vi "Node Archive and FTP File Handler.vi"() -> ()   [LabVIEW 2010]
doc: "NODE ARCHIVE & FTP is a software used to handle the file management of remote field sites using the HTI Data Logger or ATR series acoustic equipment that generates *.RAT and *.ATL files. The software monitors a specific folder on the local machine that the HTI equipment has been set up to move completed files of these types into. All other file types are ignored. The software continues to scan this file until a new file is added to the directory, on the addition of a file the NODE ARCHIVE & FTP software moves the file into an Archive directory (and if specified into a redundant Archive directory) then creates a *.ZIP version of the file and retains a copy of it in the Archive directory as well. All Zip files are then copied to a specified FTP host.\n\nNODE ARCHIVE & FTP will not try and move files for the last five minutes of an hour, or for the first five to ten minutes of the hour (based on CPU time). This is to allow the HTI hardware time to move all files at the top of the hour and avoid conflict. During the rest of the hour the software will continue to scan for new files. At any time a user can force a scan or FTP move by selecting the Manual Force FTP button or the Manual Archive Files button.\n\nNODE ARCHIVE & FTP creates an .INI file and a .CSV file in the programs application directory. The .INI file retains the last values of the file directory and FTP credentials used. The .CSV retains a history of *.ZIP files moved to the FTP and the status of their move, if there were errors or not. NODE ARCHIVE & FTP will continue to try and send the file to the FTP host until that file has completed the process with no errors. DO NOT remove or edit the .CSV file or the software will try and move all files up to the FTP again and will slow down the FTP Host."
uses:
  FTP Credintials.ctl
  <vilib>/Utility/sysdir.llb/System Directory Type.ctl
  <vilib>/Utility/error.llb/DialogType.ctl
  <vilib>/Utility/config.llb/Read Key (String).vi
  <vilib>/Utility/config.llb/Read Key (Boolean).vi
  <vilib>/Utility/config.llb/Read Key (Path).vi
  <vilib>/Utility/config.llb/Read Key (I32).vi
  <vilib>/Utility/config.llb/Write Key (Path).vi
  <vilib>/Utility/config.llb/Write Key (Boolean).vi
  <vilib>/Utility/config.llb/Write Key (String).vi
  <vilib>/Utility/config.llb/Write Key (I32).vi
  <vilib>/Utility/config.llb/NI_LVConfig.lvlib
  Aarons labview builds/telemetryCode/Utilities/NewNI_SMTPEmail Folder/NewNI_SMTPEmail.lvlib
panel:
  in  "Time DaY":timestamp
  in  "Top level Tabs":T1(tab)
  in  "ShutDown":bool
  out "Status File move":bool caption="Archiving"
  out "Status FTP move":bool caption="FTP In Progress"
  in  "Manual FTP":bool
  in  "Manual Archive":bool
  in  "FTP Creds":T2 {"FTP Timeout (S)" min=0 max=300 step=1}
  in  "Archive Location 2":path caption="(Optional) External Directory To Archive *.RAT files"
  in  "Archive Location":path=path "C:/Archive" caption="Directory To Archive *.RAT files"
  in  "Rats Location":path=path "C:/Incoming" caption="Directory To Find *.RAT files"
  in  "Ping FTP Host":bool=TRUE
  in  "Ping Node 2":bool=TRUE
  in  "Ping Node 1":bool=TRUE
  out "Node 2 Response":bool
  in  "AddressNode2":string="www.google.com" caption="Address of Node 2 to Ping"
  out "FTP Response":bool
  out "Node1 Response":bool
  in  "recipients":string[](array[string])=["nmswyers@gmail.com"] caption="Email Recipients"
  in  "Addresshost":string="50.6.185.144" caption="Address of FTP host to Ping"
  in  "AddressNode 1":string="www.google.com" caption="Address of Node 1 to Ping"
  out "Elapsed Time (H)":dbl caption="Time to Next File \nSize Check (H)" format="%#_3f"
  out "Email Notification":T3 caption="Email Notification (From INI File)"
  # "DIRECTORY SETUP:"
  # "FTP SETUP:"
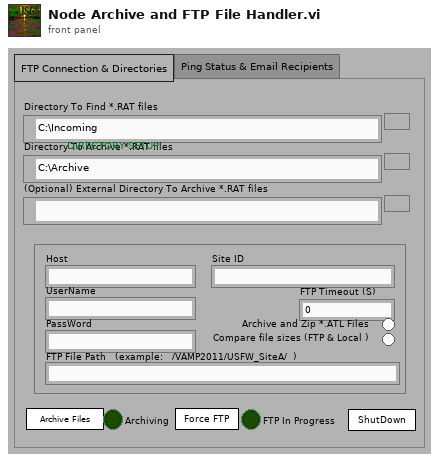
[diagram p1: front panel]
types:
  T1 = enum32{"FTP Connection & Directories", "Ping Status & Email Recipients"}
  T2 = typedef "FTP Credintials.ctl" = cluster{"Host":string, "UserName":string, "PassWord":string, "FTP File Path":string, "FTP Timeout (S)":i32, "Use ATL":bool, "Comp File Size":bool, "SITE ID":string}
  T3 = cluster{"Mail Server":string, "Return Address":string, "User Name":string, "Password":string}
  T4 = cluster{"Mail Server":string, "Return Address":string, "Email User Name":string, "Password":string}
  T5 = typedef "System Directory Type.ctl" = i32
  T6 = typedef "NI_LVConfig.lvlib/Config Data RefNum.ctl" = refnum<k1>
  T7 = typedef "DialogType.ctl" = u16
  T8 = cluster{"AddressNode 1":string, "AddressNode2":string, "Addresshost":string}
  T9 = enum16{"open", "replace", "create", "open or create", "replace or create", "replace or create with confirmation"}
  T10 = enum32{"invalid app kind", "Development System", "Run Time System", "Student Edition", "Embedded LabVIEW", "Evaluation", "Custom"}
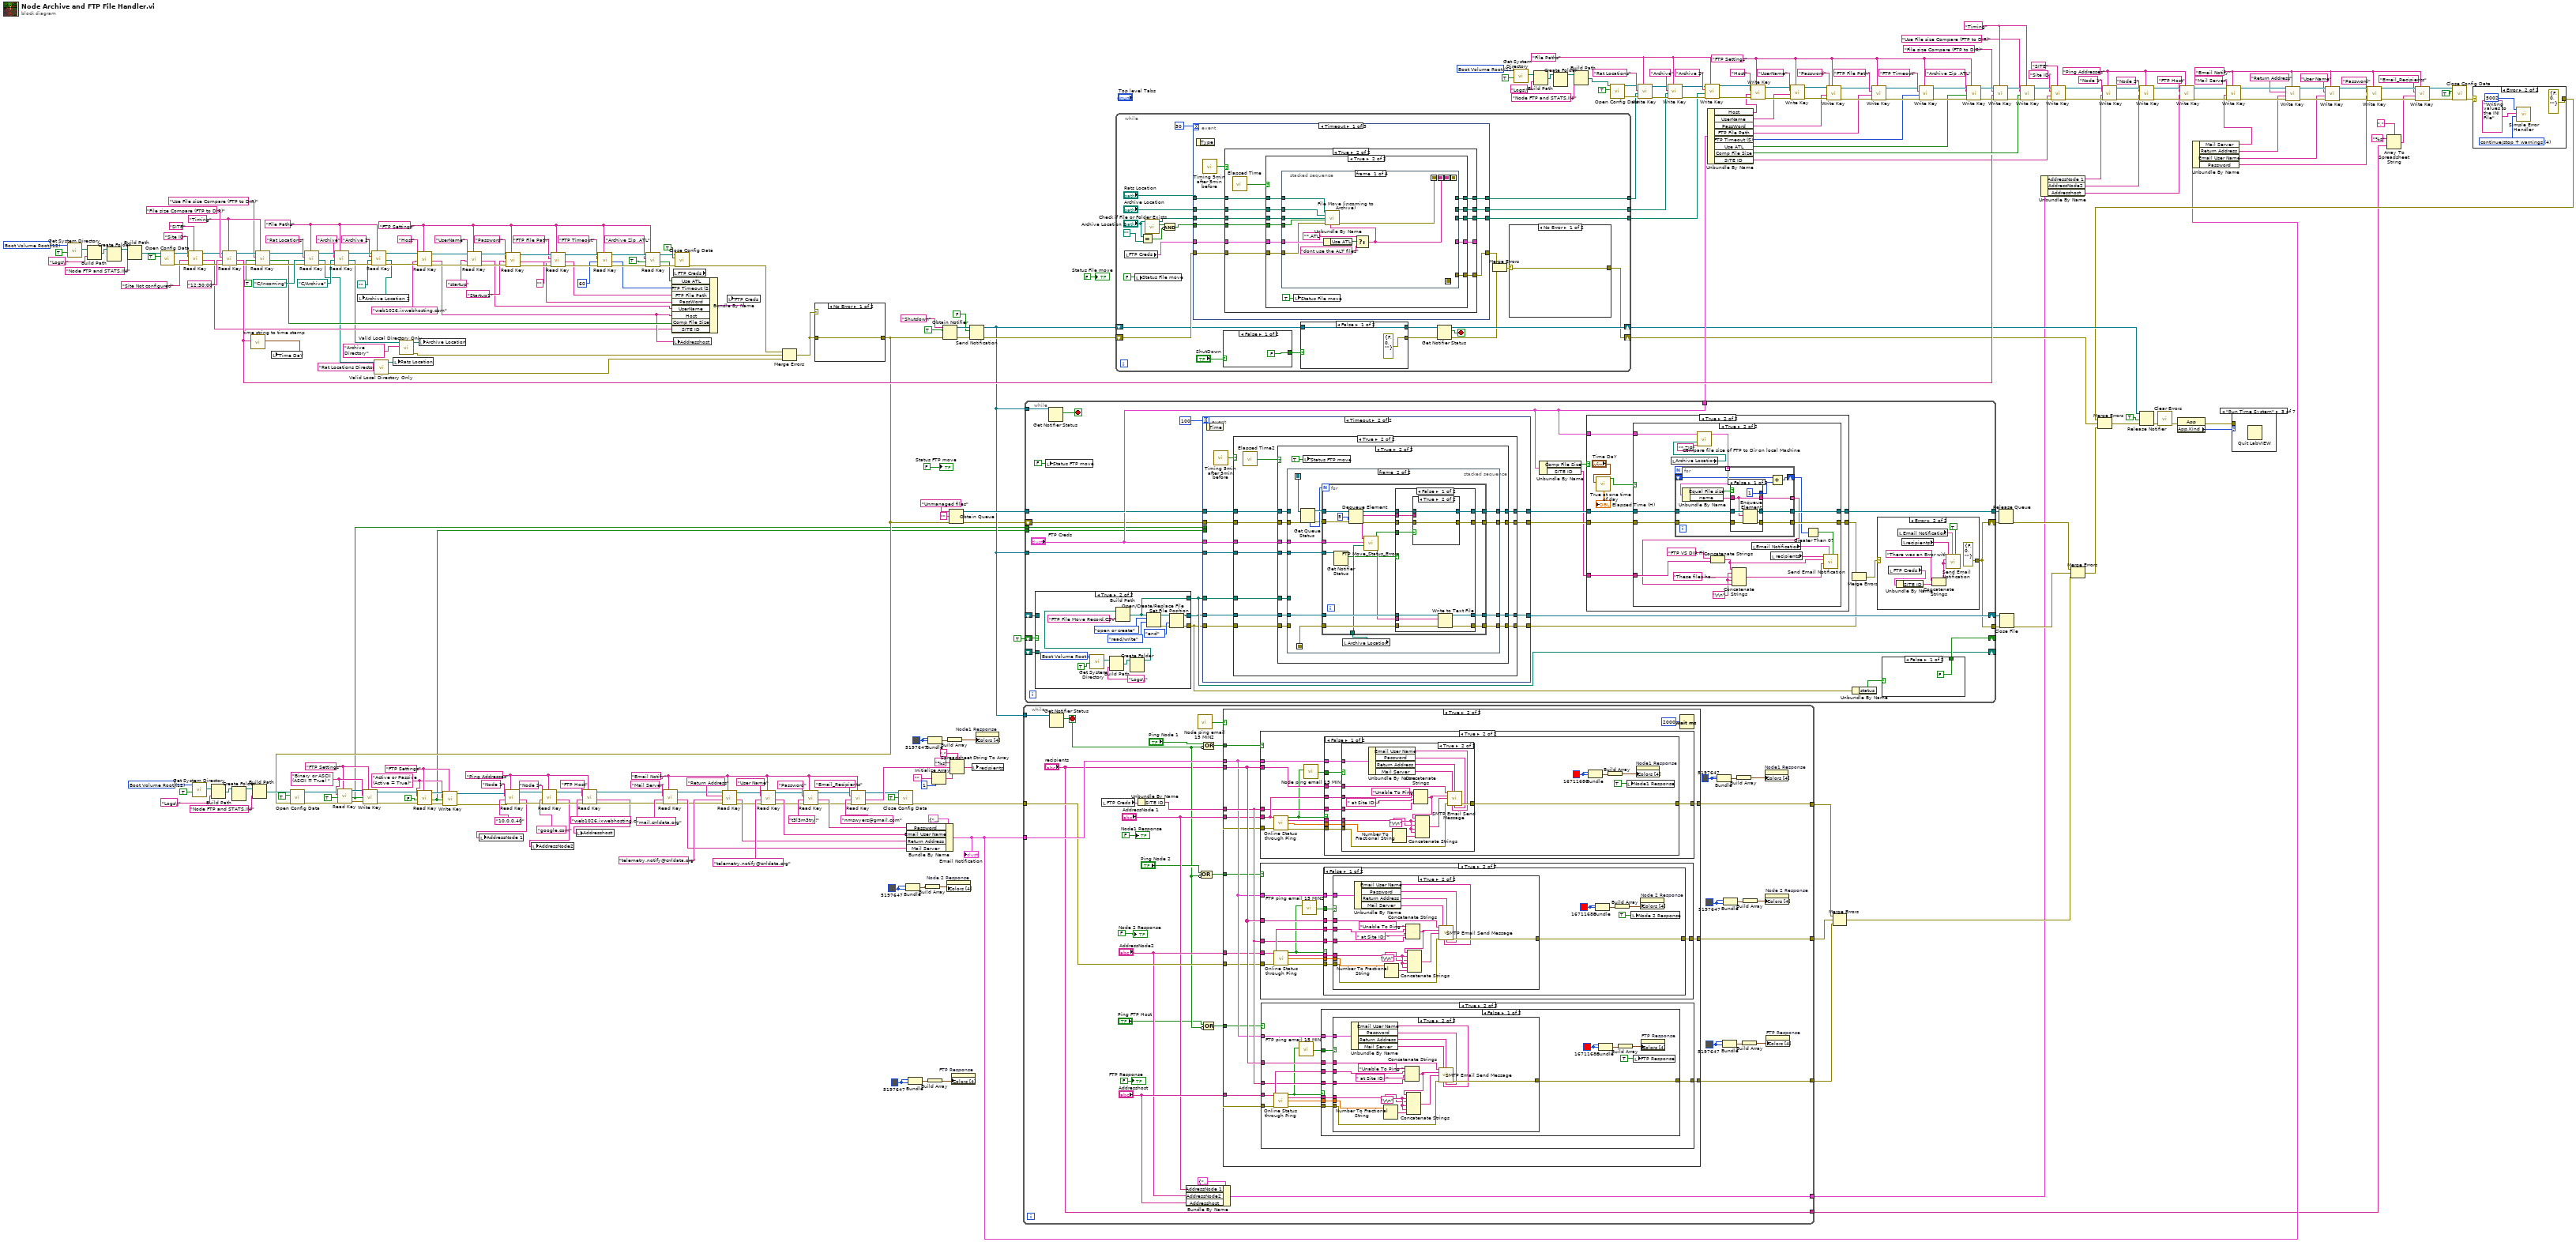
[diagram p0: block diagram]
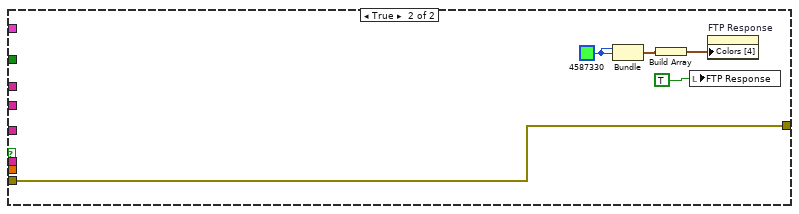
[diagram p5: hidden frame]
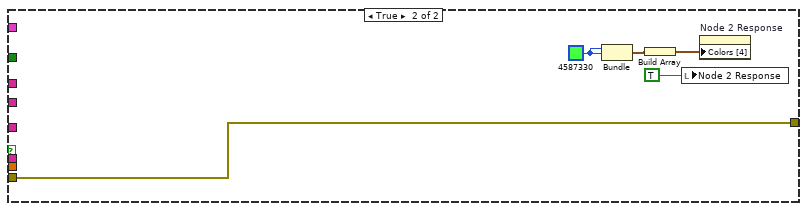
[diagram p8: hidden frame]
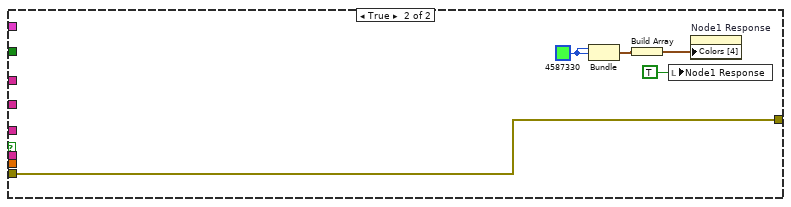
[diagram p11: hidden frame]
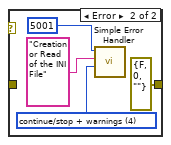
[diagram p13: hidden frame]
diagram:
  w2 = "Email Notify" ("name or relative path")
  w57 = "Binary or ASCII (ASCII = True) " ("name or relative path")
  w56 = "FTP Settings" ("name or relative path")
  w63 = "Active or Passive (Active = True)" ("name or relative path")
  w64 = "FTP Settings" ("name or relative path")
  w80 = "Ping Addresses" ("name or relative path")
  w93 = "Ping Addresses" ("name or relative path")
  w129 = u32 5197647 ("Color Box")
  w1 = "Email Notify" ("name or relative path")
  w139 = T5 12 items=["User Home"=0, "User Desktop"=1, "User Documents"=2, "User Application Data"=3, "User Preferences"=4, "User Temporary"=5, "Public Documents"=6, "Public Application Data"=7, "Public Preferences"=8, "Public Cache"=13, "System Core Libraries"=9, "System Installed Libraries"=10, "Application Files"=11, "Boot Volume Root"=12] ("system directory type")
  w155 = T5 12 items=["User Home"=0, "User Desktop"=1, "User Documents"=2, "User Application Data"=3, "User Preferences"=4, "User Temporary"=5, "Public Documents"=6, "Public Application Data"=7, "Public Preferences"=8, "Public Cache"=13, "System Core Libraries"=9, "System Installed Libraries"=10, "Application Files"=11, "Boot Volume Root"=12] ("system directory type")
  w193 = u32 5197647 ("Color Box")
  w190 = u32 5197647 ("Color Box")
  w201 = "Timing" ("name or relative path")
  w211 = "Timing" ("name or relative path")
  w266 = "FTP Settings" ("name or relative path")
  w250 = "File Paths" ("name or relative path")
  w286 = "FTP Settings" ("name or relative path")
  w304 = "File Paths" ("name or relative path")
  w306 = T5 12 items=["User Home"=0, "User Desktop"=1, "User Documents"=2, "User Application Data"=3, "User Preferences"=4, "User Temporary"=5, "Public Documents"=6, "Public Application Data"=7, "Public Preferences"=8, "Public Cache"=13, "System Core Libraries"=9, "System Installed Libraries"=10, "Application Files"=11, "Boot Volume Root"=12] ("system directory type")
  n1 = call <vilib>:"Get System Directory.vi"("create directory if not found? (F)"=TRUE, "system directory type"=w306) -> ("system directory"=w307:path)  [unwired: 9 in]
  n2 = Build Path(base path=w307, name or relative path="Logs\\" ("string")) -> (appended path=w165:path)
  n3 = Create Folder(path (use dialog)=w165) -> (created path=w164:path)  [unwired: 2 in, 2 out]
  n4 = Build Path(base path=w164, name or relative path="Node FTP and STATS.INI") -> (appended path=w162:path)
  n5 = call <vilib>:"Open Config Data.vi"("create file if necessary (T)"=TRUE, "configuration file path"=w162) -> ("error out"=w188:errorcluster, "refnum"=w187:T6)  [unwired: 7 in, 1 out]
  n6 = call-poly <vilib>:"Read Key.vi"("section"="SITE" ("name or relative path"), "error in (no error)"=w188, "default value"="Site Not configured", "key"="Site ID" ("name or relative path"), "refnum"=w187) -> ("error out"=w185:errorcluster, "value"=w181:string, "refnum out"=w186:T6)  [unwired: 3 in, 1 out]
  n7 = call <vilib>:"Get System Directory.vi"("create directory if not found? (F)"=TRUE, "system directory type"=w139) -> ("system directory"=w138:path)  [unwired: 9 in]
  n8 = Build Path(base path=w138, name or relative path="Logs\\" ("string")) -> (appended path=w144:path)
  n9 = call-poly <vilib>:"Read Key.vi"("section"=w211, "error in (no error)"=w185, "default value"="12:30:00", "key"="File size Compare (FTP to DIR)" ("name or relative path"), "refnum"=w186) -> ("error out"=w215:errorcluster, "value"=w196:string, "refnum out"=w214:T6)  [unwired: 3 in, 1 out]
  n10 = Create Folder(path (use dialog)=w144) -> (created path=w145:path)  [unwired: 2 in, 2 out]
  n11 = call "time string to time stamp.vi"("time string example(16:15:00)"=w196) -> ("time stamp"=w208:timestamp)  [unwired: 10 in]
  n12 = Build Path(base path=w145, name or relative path="Node FTP and STATS.INI") -> (appended path=w147:path)
  n13 = call-poly <vilib>:"Read Key.vi"("section"=w211, "error in (no error)"=w215, "default value"=TRUE ("create file if necessary (T)"), "key"="Use File size Compare (FTP to DIR)" ("name or relative path"), "refnum"=w214) -> ("error out"=w212:errorcluster, "value"=w198:bool, "refnum out"=w213:T6)  [unwired: 3 in, 1 out]
  n14 = local write "Time DaY"(w208) -> ()
  n15 = call-poly <vilib>:"Read Key.vi"("section"=w304, "error in (no error)"=w212, "default value"=path "C:/Incoming", "key"="Rat Locations" ("name or relative path"), "refnum"=w213) -> ("error out"=w311:errorcluster, "value"=w174:path, "refnum out"=w312:T6)  [unwired: 3 in, 1 out]
  n16 = call-poly <vilib>:"Read Key.vi"("section"=w304, "error in (no error)"=w311, "default value"=path "C:/Archive", "key"="Archive" ("name or relative path"), "refnum"=w312) -> ("error out"=w309:errorcluster, "value"=w170:path, "refnum out"=w310:T6)  [unwired: 3 in, 1 out]
  n17 = call-poly <vilib>:"Read Key.vi"("section"=w304, "error in (no error)"=w309, "default value"=path "", "key"="Archive 2" ("name or relative path"), "refnum"=w310) -> ("error out"=w300:errorcluster, "value"=w161:path, "refnum out"=w293:T6)  [unwired: 3 in, 1 out]
  n18 = local write "Archive Location 2"(w161) -> ()
  n19 = call "Valid Local Directory Only.vi"("Directory ref"="Rat Locations Directory", "Path input"=w174) -> ("error out"=w149:errorcluster, "Path output"=w172:path)  [unwired: 8 in]
  n20 = local write "Rats Location"(w172) -> ()
  n21 = call "Valid Local Directory Only.vi"("Directory ref"="Archive Directory", "Path input"=w170) -> ("error out"=w150:errorcluster, "Path output"=w169:path)  [unwired: 8 in]
  n22 = call-poly <vilib>:"Read Key.vi"("section"=w286, "error in (no error)"=w300, "default value"="web1026.ixwebhosting.com" ("name or relative path"), "key"="Host" ("name or relative path"), "refnum"=w293) -> ("error out"=w299:errorcluster, "value"=w194:string, "refnum out"=w292:T6)  [unwired: 3 in, 1 out]
  n23 = local write "Archive Location"(w169) -> ()
  n24 = call-poly <vilib>:"Read Key.vi"("section"=w286, "error in (no error)"=w299, "default value"="startup" ("name or relative path"), "key"="UserName" ("name or relative path"), "refnum"=w292) -> ("error out"=w298:errorcluster, "value"=w230:string, "refnum out"=w291:T6)  [unwired: 3 in, 1 out]
  n25 = call-poly <vilib>:"Read Key.vi"("section"=w286, "error in (no error)"=w298, "default value"="Startup1" ("name or relative path"), "key"="Password" ("name or relative path"), "refnum"=w291) -> ("error out"=w297:errorcluster, "value"=w231:string, "refnum out"=w290:T6)  [unwired: 3 in, 1 out]
  n26 = call-poly <vilib>:"Read Key.vi"("section"=w286, "error in (no error)"=w297, "default value"="" ("name or relative path"), "key"="FTP File Path" ("name or relative path"), "refnum"=w290) -> ("error out"=w296:errorcluster, "value"=w232:string, "refnum out"=w289:T6)  [unwired: 3 in, 1 out]
  n27 = call-poly <vilib>:"Read Key.vi"("section"=w286, "error in (no error)"=w296, "default value"=60, "key"="FTP Timeout" ("name or relative path"), "refnum"=w289) -> ("error out"=w295:errorcluster, "value"=w67:i32, "refnum out"=w288:T6)  [unwired: 3 in, 1 out]
  n28 = call-poly <vilib>:"Read Key.vi"("section"=w286, "error in (no error)"=w295, "default value"=TRUE, "key"="Archive Zip .ATL" ("name or relative path"), "refnum"=w288) -> ("error out"=w294:errorcluster, "value"=w233:bool, "refnum out"=w287:T6)  [unwired: 3 in, 1 out]
  n29 = local read "FTP Creds"() -> (w234:T2)
  n30 = Bundle By Name(cluster=w234, "Use ATL"=w233, "FTP Timeout (S)"=w67, "FTP File Path"=w232, "PassWord"=w231, "UserName"=w230, "Host"=w194, "Comp File Size"=w198, "SITE ID"=w181) -> (w235:T2)
  n31 = local write "Addresshost"(w194) -> ()
  n32 = call <vilib>:"Close Config Data.vi"("error in (no error)"=w294, "write file if changed (T)"=TRUE, "refnum"=w287) -> ("error out"=w151:errorcluster)  [unwired: 7 in, 1 out]
  n33 = local write "FTP Creds"(w235) -> ()
  n34 = Merge Errors(w151, w150, w149) -> (w152:errorcluster)
  n35 = case shown="No Error" w152 {
    tunnel: w152 -> [w314 _]
    tunnel: [w314 errorcluster {"status"=FALSE, "code"=0, "source"=""} ("error out")] -> w104
    frame No Error {
    }
    frame Error {
      w318 = T7 4 items=["no dialog", "OK message", "continue or stop message", "OK message + warnings", "continue/stop + warnings"] ("type of dialog (OK msg:1)")
      n36 = call <vilib>:"Simple Error Handler.vi"("error code (no error:0)"=5001, "error source (\" \")"="Creation or Read of the INI File" ("error source (\" \")"), "type of dialog (OK msg:1)"=w318) -> ()  [unwired: 2 in, 5 out]
    }
  }
  n37 = call <vilib>:"Open Config Data.vi"("error in (no error)"=w104, "create file if necessary (T)"=TRUE, "configuration file path"=w147) -> ("error out"=w53:errorcluster, "refnum"=w54:T6)  [unwired: 6 in, 1 out]
  n38 = call-poly <vilib>:"Read Key.vi"("section"=w56, "error in (no error)"=w53, "default value"=TRUE, "key"=w57, "refnum"=w54) -> ("error out"=w52:errorcluster, "value"=w49:bool, "refnum out"=w55:T6)  [unwired: 3 in, 1 out]
  n39 = call-poly <vilib>:"Write Key.vi"("section"=w56, "error in (no error)"=w52, "value"=w49, "key"=w57, "refnum"=w55) -> ("error out"=w51:errorcluster, "refnum out"=w50:T6)  [unwired: 4 in, 1 out]
  n40 = call-poly <vilib>:"Read Key.vi"("section"=w64, "error in (no error)"=w51, "default value"=FALSE, "key"=w63, "refnum"=w50) -> ("error out"=w66:errorcluster, "value"=w59:bool, "refnum out"=w65:T6)  [unwired: 3 in, 1 out]
  n41 = call-poly <vilib>:"Write Key.vi"("section"=w64, "error in (no error)"=w66, "value"=w59, "key"=w63, "refnum"=w65) -> ("error out"=w60:errorcluster, "refnum out"=w61:T6)  [unwired: 4 in, 1 out]
  n42 = call-poly <vilib>:"Read Key.vi"("section"=w93, "error in (no error)"=w60, "default value"="10.0.0.40", "key"="Node 1" ("Mail Server"), "refnum"=w61) -> ("error out"=w91:errorcluster, "value"=w86:string, "refnum out"=w92:T6)  [unwired: 3 in, 1 out]
  n43 = local write "AddressNode 1"(w86) -> ()
  n44 = call-poly <vilib>:"Read Key.vi"("section"=w93, "error in (no error)"=w91, "default value"="google.com", "key"="Node 2" ("Mail Server"), "refnum"=w92) -> ("error out"=w90:errorcluster, "value"=w85:string, "refnum out"=w89:T6)  [unwired: 3 in, 1 out]
  n45 = local write "AddressNode2"(w85) -> ()
  n46 = call-poly <vilib>:"Read Key.vi"("section"=w93, "error in (no error)"=w90, "default value"="web1026.ixwebhosting.com", "key"="FTP Host" ("Mail Server"), "refnum"=w89) -> ("error out"=w87:errorcluster, "value"=w84:string, "refnum out"=w88:T6)  [unwired: 3 in, 1 out]
  n47 = local write "Addresshost"(w84) -> ()
  n48 = call-poly <vilib>:"Read Key.vi"("section"=w1, "error in (no error)"=w87, "default value"="mail.crrldata.org", "key"="Mail Server" ("Mail Server"), "refnum"=w88) -> ("error out"=w47:errorcluster, "value"=w118:string, "refnum out"=w46:T6)  [unwired: 3 in, 1 out]
  n49 = call-poly <vilib>:"Read Key.vi"("section"=w1, "error in (no error)"=w47, "default value"="telemetry.notify@crrldata.org", "key"="Return Address" ("Return Address"), "refnum"=w46) -> ("error out"=w45:errorcluster, "value"=w119:string, "refnum out"=w42:T6)  [unwired: 3 in, 1 out]
  n50 = call-poly <vilib>:"Read Key.vi"("section"=w1, "error in (no error)"=w45, "default value"="telemetry.notify@crrldata.org", "key"="User Name" ("Email User Name"), "refnum"=w42) -> ("error out"=w44:errorcluster, "value"=w120:string, "refnum out"=w43:T6)  [unwired: 3 in, 1 out]
  n51 = call-poly <vilib>:"Read Key.vi"("section"=w1, "error in (no error)"=w44, "default value"="t3l3m3try!", "key"="Password" ("Password"), "refnum"=w43) -> ("error out"=w33:errorcluster, "value"=w121:string, "refnum out"=w34:T6)  [unwired: 3 in, 1 out]
  n52 = call-poly <vilib>:"Read Key.vi"("section"=w1, "error in (no error)"=w33, "default value"="nmswyers@gmail.com", "key"="Email_Recipients" ("Password"), "refnum"=w34) -> ("error out"=w30:errorcluster, "value"=w32:string, "refnum out"=w31:T6)  [unwired: 3 in, 1 out]
  n53 = call <vilib>:"Close Config Data.vi"("error in (no error)"=w30, "write file if changed (T)"=TRUE, "refnum"=w31) -> ("error out"=w132:errorcluster)  [unwired: 7 in, 1 out]
  n54 = Bundle("Color Box"=w193, "Color Box"=w193) -> (w192:cluster{"Color Box":u32, "Color Box":u32})  [unwired: 1 in]
  n55 = Bundle By Name(cluster=T4 {"Mail Server"="Mail Server", "Return Address"="Return Address", "Email User Name"="User Name", "Password"="Password"} ("input cluster"), "Password"=w121, "Email User Name"=w120, "Return Address"=w119, "Mail Server"=w118) -> (w11:T4)
  "Email Notification" <- w11
  n56 = Bundle("Color Box"=w129, "Color Box"=w129) -> (w130:cluster{"Color Box":u32, "Color Box":u32})  [unwired: 1 in]
  n57 = Build Array(w192) -> (w128:cluster{"Color Box":u32, "Color Box":u32}[])
  n58 = Bundle("Color Box"=w190, "Color Box"=w190) -> (w189:cluster{"Color Box":u32, "Color Box":u32})  [unwired: 1 in]
  n59 = Build Array(w130) -> (w131:cluster{"Color Box":u32, "Color Box":u32}[])
  n60 = Initialize Array("", 1 ("dimension size")) -> (w41:string[])
  n61 = Obtain Notifier(name (unnamed)="Shutdown", notification data type=TRUE, error in (no error)=w104) -> (notifier out=w115:refnum<notifier>, error out=w113:errorcluster)  [unwired: 1 in, 1 out]
  n62 = property on="Node 2 Response" class="Bool (strict)"("Colors [4]"=w128) -> ()  [unwired: 2 in, 2 out]
  n63 = Build Array(w189) -> (w191:cluster{"Color Box":u32, "Color Box":u32}[])
  n64 = Obtain Queue(name (unnamed)="Unmanaged files", element data type="" ("name (unnamed)"), error in (no error)=w104) -> (queue out=w222:refnum<queue>, error out=w48:errorcluster)  [unwired: 2 in, 1 out]
  n65 = Spreadsheet String To Array(delimiter (Tab)=",", format string="%s", spreadsheet string=w32, array type (2D Dbl)=w41) -> (array=w29:string[])
  n66 = property on="FTP Response" class="Bool (strict)"("Colors [4]"=w131) -> ()  [unwired: 2 in, 2 out]
  n67 = Send Notification(notification=FALSE, notifier=w115, error in (no error)=w113) -> (notifier out=w68:refnum<notifier>, error out=w112:errorcluster)
  n68 = local write "recipients"(w29) -> ()
  n69 = property on="Node1 Response" class="Bool (strict)"("Colors [4]"=w191) -> ()  [unwired: 2 in, 2 out]
  n70 = while {
    tunnel: w132 -> [w342]
    tunnel: [w349] -> w168
    tunnel: w11 -> [w344]
    tunnel: [w346] -> w127
    tunnel: [w345] -> w126
    tunnel: w68 -> [w343]
    tunnel: [w337] -> w83
    tunnel: ["recipients"] -> w6
    stop <- w331 stop-if-true
    w323 = u32 5197647 ("Color Box")
    w324 = u32 5197647 ("Color Box")
    w328 = u32 5197647 ("Color Box")
    n71 = Get Notifier Status(notifier=w343) -> (current notification=w331:bool)  [unwired: 1 in, 4 out]
    n72 = local read "FTP Creds"() -> (w350:T2)
    n73 = Unbundle By Name(w350) -> ("SITE ID"=w347:string)
    n74 = Bundle By Name(cluster=T8 {"AddressNode 1"="www.google.com", "AddressNode2"="www.google.com", "Addresshost"="50.6.185.144"} ("input cluster"), "AddressNode 1"="AddressNode 1", "AddressNode2"="AddressNode2", "Addresshost"="Addresshost") -> (w337:T8)
    n75 = call "Node ping email 15 MIN2"() -> ("Time has Elapsed"=w320:bool)  [unwired: 12 in, 7 out]
    n76 = Compound Arithmetic op=OR("Ping Node 2", invert w331) -> (w334:bool)
    n77 = Compound Arithmetic op=OR("Ping Node 1", invert w331) -> (w336:bool)
    n78 = Compound Arithmetic op=OR("Ping FTP Host", invert w331) -> (w332:bool)
    n79 = case shown="True" w320 {
      tunnel: [w353 w367] -> w349
      tunnel: "recipients" -> [_ w366]
      tunnel: w347 -> [_ w365]
      tunnel: [w353 w364] -> w346
      tunnel: [w353 w363] -> w345
      tunnel: w344 -> [_ w362]
      tunnel: w342 -> [w353 w361]
      tunnel: "Addresshost" -> [_ w360]
      tunnel: "AddressNode2" -> [_ w359]
      tunnel: "AddressNode 1" -> [_ w358]
      tunnel: w336 -> [_ w357]
      tunnel: w334 -> [_ w356]
      tunnel: w332 -> [_ w355]
      frame False {
      }
      frame True {
        n80 = case shown="True" w357 {
          tunnel: w358 -> [_ w475]
          tunnel: [w466 w473] -> w367
          tunnel: w366 -> [_ w472]
          tunnel: w361 -> [w466 w471]
          tunnel: w365 -> [_ w470]
          tunnel: w362 -> [_ w469]
          frame False {
          }
          frame True {
            n81 = call "Online Status through Ping.vi"("AddressToPing"=w475, "error in (no error)"=w471) -> ("Connection?"=w467:bool, "Standard Output"=w477:string, "% Recieved"=w476:dbl, "error out"=w474:errorcluster)  [unwired: 9 in, 1 out]
            n82 = call "Node ping email 15 MIN"("Reset"=w467) -> ("Time has Elapsed"=w468:bool)  [unwired: 11 in, 7 out]
            n83 = case shown="False" w467 {
              tunnel: w477 -> [w490 _]
              tunnel: w476 -> [w489 _]
              tunnel: w472 -> [w488 _]
              tunnel: w475 -> [w487 _]
              tunnel: w470 -> [w482 _]
              tunnel: w474 -> [w481 w510]
              tunnel: [w480 w510] -> w473
              tunnel: w469 -> [w479 _]
              tunnel: w468 -> [w478 _]
              frame False {
                w485 = u32 16711680 ("Color Box")
                n84 = case shown="True" w478 {
                  tunnel: w490 -> [_ w501]
                  tunnel: w489 -> [_ w504]
                  tunnel: w488 -> [_ w503]
                  tunnel: w487 -> [_ w502]
                  tunnel: w482 -> [_ w499]
                  tunnel: w481 -> [w491 w498]
                  tunnel: [w491 w497] -> w480
                  tunnel: w479 -> [_ w496]
                  frame False {
                  }
                  frame True {
                    w508 = "\r\n"
                    n85 = Unbundle By Name(w496) -> ("Email User Name"=w492:string, "Password"=w493:string, "Return Address"=w494:string, "Mail Server"=w495:string)
                    n86 = Number To Fractional String(number=w504) -> (F-format string=w507:string)  [unwired: 3 in]
                    n87 = Concatenate Strings("Unable To Ping " ("subject ([No Subject])"), w502, " at Site ID: " ("string"), w499) -> (w506:string)
                    n88 = Concatenate Strings(w506, w508, w501, w508, w508, w507) -> (w505:string)
                    n89 = call "SMTP Email Send Message.vi"("recipients"=w503, "mail server"=w495, "return address"=w494, "subject ([No Subject])"=w506, "message"=w505, "error in (no error)"=w498, "username"=w492, "password"=w493) -> ("error out"=w497:errorcluster)  [unwired: 7 out]
                  }
                }
                n90 = Bundle("Color Box"=w485, "Color Box"=w485) -> (w484:cluster{"Color Box":u32, "Color Box":u32})  [unwired: 1 in]
                n91 = Build Array(w484) -> (w486:cluster{"Color Box":u32, "Color Box":u32}[])
                n92 = local write "Node1 Response"(TRUE ("Node Responding")) -> ()
                n93 = property on="Node1 Response" class="Bool (strict)"("Colors [4]"=w486) -> ()  [unwired: 2 in, 2 out]
              }
              frame True {
                w513 = u32 4587330 ("Color Box")
                n94 = Bundle("Color Box"=w513, "Color Box"=w513) -> (w514:cluster{"Color Box":u32, "Color Box":u32})  [unwired: 1 in]
                n95 = Build Array(w514) -> (w512:cluster{"Color Box":u32, "Color Box":u32}[])
                n96 = local write "Node1 Response"(TRUE ("Node Responding")) -> ()
                n97 = property on="Node1 Response" class="Bool (strict)"("Colors [4]"=w512) -> ()  [unwired: 2 in, 2 out]
              }
            }
          }
        }
        n98 = case shown="True" w356 {
          tunnel: w359 -> [_ w425]
          tunnel: w366 -> [_ w424]
          tunnel: w361 -> [w417 w423]
          tunnel: w365 -> [_ w422]
          tunnel: [w417 w421] -> w364
          tunnel: w362 -> [_ w420]
          frame False {
          }
          frame True {
            n99 = call "Online Status through Ping.vi"("AddressToPing"=w425, "error in (no error)"=w423) -> ("Connection?"=w418:bool, "Standard Output"=w427:string, "% Recieved"=w426:dbl, "error out"=w428:errorcluster)  [unwired: 9 in, 1 out]
            n100 = call "FTP ping email 15 MIN2"("Reset"=w418) -> ("Time has Elapsed"=w419:bool)  [unwired: 11 in, 7 out]
            n101 = case shown="False" w418 {
              tunnel: w427 -> [w441 _]
              tunnel: w426 -> [w440 _]
              tunnel: w424 -> [w439 _]
              tunnel: w425 -> [w438 _]
              tunnel: w422 -> [w435 _]
              tunnel: w428 -> [w434 w463]
              tunnel: [w433 w463] -> w421
              tunnel: w420 -> [w430 _]
              tunnel: w419 -> [w429 _]
              frame False {
                w437 = u32 16711680 ("Color Box")
                n102 = case shown="True" w429 {
                  tunnel: w441 -> [_ w452]
                  tunnel: w440 -> [_ w455]
                  tunnel: w439 -> [_ w454]
                  tunnel: w438 -> [_ w453]
                  tunnel: w435 -> [_ w450]
                  tunnel: w434 -> [w442 w449]
                  tunnel: [w442 w448] -> w433
                  tunnel: w430 -> [_ w447]
                  frame False {
                  }
                  frame True {
                    w459 = "\r\n"
                    n103 = Unbundle By Name(w447) -> ("Email User Name"=w443:string, "Password"=w444:string, "Return Address"=w445:string, "Mail Server"=w446:string)
                    n104 = Number To Fractional String(number=w455) -> (F-format string=w458:string)  [unwired: 3 in]
                    n105 = Concatenate Strings("Unable To Ping " ("subject ([No Subject])"), w453, " at Site ID: " ("string"), w450) -> (w457:string)
                    n106 = Concatenate Strings(w457, w459, w452, w459, w459, w458) -> (w456:string)
                    n107 = call "SMTP Email Send Message.vi"("recipients"=w454, "mail server"=w446, "return address"=w445, "subject ([No Subject])"=w457, "message"=w456, "error in (no error)"=w449, "username"=w443, "password"=w444) -> ("error out"=w448:errorcluster)  [unwired: 7 out]
                  }
                }
                n108 = Bundle("Color Box"=w437, "Color Box"=w437) -> (w436:cluster{"Color Box":u32, "Color Box":u32})  [unwired: 1 in]
                n109 = Build Array(w436) -> (w432:cluster{"Color Box":u32, "Color Box":u32}[])
                n110 = local write "Node 2 Response"(TRUE ("FTP Responding")) -> ()
                n111 = property on="Node 2 Response" class="Bool (strict)"("Colors [4]"=w432) -> ()  [unwired: 2 in, 2 out]
              }
              frame True {
                w465 = u32 4587330 ("Color Box")
                n112 = Bundle("Color Box"=w465, "Color Box"=w465) -> (w464:cluster{"Color Box":u32, "Color Box":u32})  [unwired: 1 in]
                n113 = Build Array(w464) -> (w462:cluster{"Color Box":u32, "Color Box":u32}[])
                n114 = local write "Node 2 Response"(TRUE) -> ()
                n115 = property on="Node 2 Response" class="Bool (strict)"("Colors [4]"=w462) -> ()  [unwired: 2 in, 2 out]
              }
            }
          }
        }
        n116 = case shown="True" w355 {
          tunnel: w360 -> [_ w379]
          tunnel: w366 -> [_ w375]
          tunnel: w361 -> [w368 w374]
          tunnel: w365 -> [_ w373]
          tunnel: [w368 w372] -> w363
          tunnel: w362 -> [_ w371]
          frame False {
          }
          frame True {
            n117 = call "Online Status through Ping.vi"("AddressToPing"=w379, "error in (no error)"=w374) -> ("Connection?"=w369:bool, "Standard Output"=w377:string, "% Recieved"=w378:dbl, "error out"=w376:errorcluster)  [unwired: 9 in, 1 out]
            n118 = call "FTP ping email 15 MIN"("Reset"=w369) -> ("Time has Elapsed"=w370:bool)  [unwired: 11 in, 7 out]
            n119 = case shown="False" w369 {
              tunnel: w377 -> [w392 _]
              tunnel: w378 -> [w391 _]
              tunnel: w375 -> [w390 _]
              tunnel: w379 -> [w389 _]
              tunnel: w373 -> [w384 _]
              tunnel: w376 -> [w383 w412]
              tunnel: [w382 w412] -> w372
              tunnel: w371 -> [w381 _]
              tunnel: w370 -> [w380 _]
              frame False {
                w388 = u32 16711680 ("Color Box")
                n120 = case shown="True" w380 {
                  tunnel: w392 -> [_ w403]
                  tunnel: w391 -> [_ w406]
                  tunnel: w390 -> [_ w405]
                  tunnel: w389 -> [_ w404]
                  tunnel: w384 -> [_ w401]
                  tunnel: w383 -> [w393 w400]
                  tunnel: [w393 w399] -> w382
                  tunnel: w381 -> [_ w398]
                  frame False {
                  }
                  frame True {
                    w410 = "\r\n"
                    n121 = Unbundle By Name(w398) -> ("Email User Name"=w394:string, "Password"=w395:string, "Return Address"=w396:string, "Mail Server"=w397:string)
                    n122 = Number To Fractional String(number=w406) -> (F-format string=w409:string)  [unwired: 3 in]
                    n123 = Concatenate Strings("Unable To Ping " ("subject ([No Subject])"), w404, " at Site ID: " ("string"), w401) -> (w408:string)
                    n124 = Concatenate Strings(w408, w410, w403, w410, w410, w409) -> (w407:string)
                    n125 = call "SMTP Email Send Message.vi"("recipients"=w405, "mail server"=w397, "return address"=w396, "subject ([No Subject])"=w408, "message"=w407, "error in (no error)"=w400, "username"=w394, "password"=w395) -> ("error out"=w399:errorcluster)  [unwired: 7 out]
                  }
                }
                n126 = Bundle("Color Box"=w388, "Color Box"=w388) -> (w387:cluster{"Color Box":u32, "Color Box":u32})  [unwired: 1 in]
                n127 = Build Array(w387) -> (w386:cluster{"Color Box":u32, "Color Box":u32}[])
                n128 = local write "FTP Response"(TRUE ("FTP Responding")) -> ()
                n129 = property on="FTP Response" class="Bool (strict)"("Colors [4]"=w386) -> ()  [unwired: 2 in, 2 out]
              }
              frame True {
                w415 = u32 4587330 ("Color Box")
                n130 = Bundle("Color Box"=w415, "Color Box"=w415) -> (w414:cluster{"Color Box":u32, "Color Box":u32})  [unwired: 1 in]
                n131 = Build Array(w414) -> (w413:cluster{"Color Box":u32, "Color Box":u32}[])
                n132 = local write "FTP Response"(TRUE) -> ()
                n133 = property on="FTP Response" class="Bool (strict)"("Colors [4]"=w413) -> ()  [unwired: 2 in, 2 out]
              }
            }
          }
        }
        n134 = Wait (ms)(milliseconds to wait=u32 2000) -> ()  [unwired: 1 out]
      }
    }
    n135 = Bundle("Color Box"=w328, "Color Box"=w328) -> (w329:cluster{"Color Box":u32, "Color Box":u32})  [unwired: 1 in]
    n136 = Bundle("Color Box"=w324, "Color Box"=w324) -> (w325:cluster{"Color Box":u32, "Color Box":u32})  [unwired: 1 in]
    n137 = Bundle("Color Box"=w323, "Color Box"=w323) -> (w322:cluster{"Color Box":u32, "Color Box":u32})  [unwired: 1 in]
    n138 = Build Array(w329) -> (w327:cluster{"Color Box":u32, "Color Box":u32}[])
    n139 = Build Array(w325) -> (w326:cluster{"Color Box":u32, "Color Box":u32}[])
    n140 = Build Array(w322) -> (w321:cluster{"Color Box":u32, "Color Box":u32}[])
    n141 = property on="Node1 Response" class="Bool (strict)"("Colors [4]"=w327) -> ()  [unwired: 2 in, 2 out]
    n142 = property on="Node 2 Response" class="Bool (strict)"("Colors [4]"=w321) -> ()  [unwired: 2 in, 2 out]
    n143 = property on="FTP Response" class="Bool (strict)"("Colors [4]"=w326) -> ()  [unwired: 2 in, 2 out]
    "Node1 Response" <- FALSE
    "FTP Response" <- FALSE ("FTP Responding")
    "Node 2 Response" <- FALSE ("FTP Responding")
  }
  n144 = while {
    tunnel: w222 -> [w540]
    tunnel: [w530] -> w206
    shift-right: [w534] -> _
    shift-left: TRUE ("create directory if not found? (F)") -> [w537]
    shift-right: [w541] -> w225
    shift-left: _ -> [w536]
    shift-right: [w533] -> _
    shift-left: _ -> [w532]
    tunnel: ["FTP Creds"] -> w175
    tunnel: w68 -> [w522]
    tunnel: [w519] -> w100
    shift-right: [w519] -> w101
    shift-left: w48 -> [w515]
    tunnel: w68 -> [w518]
    tunnel: w59 -> [w517]
    tunnel: w49 -> [w516]
    stop <- w521 stop-if-true
    n145 = case shown="True" w537 {
      tunnel: w536 -> [w608 _]
      tunnel: [errorcluster {"status"=FALSE, "code"=0, "source"=""} ("error out") w613] -> w523
      tunnel: [w609 w612] -> w533
      tunnel: w532 -> [w609 _]
      tunnel: [w608 w611] -> w524
      frame False {
      }
      frame True {
        w619 = T5 12 items=["User Home"=0, "User Desktop"=1, "User Documents"=2, "User Application Data"=3, "User Preferences"=4, "User Temporary"=5, "Public Documents"=6, "Public Application Data"=7, "Public Preferences"=8, "Public Cache"=13, "System Core Libraries"=9, "System Installed Libraries"=10, "Application Files"=11, "Boot Volume Root"=12] ("system directory type")
        n146 = call <vilib>:"Get System Directory.vi"("create directory if not found? (F)"=TRUE, "system directory type"=w619) -> ("system directory"=w620:path)  [unwired: 9 in]
        n147 = Build Path(base path=w620, name or relative path="Logs\\" ("string")) -> (appended path=w616:path)
        n148 = Create Folder(path (use dialog)=w616) -> (created path=w615:path)  [unwired: 2 in, 2 out]
        n149 = Build Path(base path=w615, name or relative path="FTP File Move Record.CSV") -> (appended path=w612:path)
        n150 = Open/Create/Replace File(file path (use dialog)=w612, operation (0:open)=T9."open or create", access (0:read/write)=enum16{"read/write", "read-only", "write-only"}."read/write") -> (refnum out=w623:refnum<file>, error out=w624:errorcluster)  [unwired: 3 in, 1 out]
        n151 = Set File Position(refnum=w623, from (0:start)=enum16{"start", "end", "current"}."end", error in=w624) -> (refnum out=w611:refnum<file>, error out=w613:errorcluster)  [unwired: 1 in]
      }
    }
    n152 = local write "Status FTP move"(FALSE ("Status FTP move")) -> ()
    n153 = Get Notifier Status(notifier=w522) -> (current notification=w521:bool)  [unwired: 1 in, 4 out]
    n154 = event shown="[1] Timeout" {
      selector: _ -> [_ _]
      dyn-events: _ -> [_ _]
      timeout: 100 -> [_ _]
      tunnel: [w639 w729] -> w541
      tunnel: w540 -> [w638 w728]
      tunnel: [w637 w727] -> w531
      tunnel: w515 -> [w636 w726]
      tunnel: [w635 w725] -> w529
      tunnel: [w634 w724] -> w539
      tunnel: w524 -> [w632 w722]
      tunnel: w523 -> [w631 w721]
      tunnel: w533 -> [w630 w720]
      tunnel: "FTP Creds" -> [w629 w719]
      tunnel: w518 -> [w628 w718]
      tunnel: w517 -> [w627 _]
      tunnel: w516 -> [w626 _]
      event "Manual FTP": Value Change {
        n155 = event-data() -> ()  [unwired: 1 in, 1 out]
        n156 = local write "Status FTP move"(TRUE ("Status FTP move")) -> ()
        n157 = stacked-sequence {
          seq-local: [w646 _] -> [_ w670]
          seq-local: [w645 _] -> [_ w669]
          tunnel: [_ w673] -> w639
          tunnel: w638 -> [w647 _]
          tunnel: [_ w671] -> w637
          tunnel: w636 -> [w643 w666]
          tunnel: [_ w664] -> w635
          tunnel: [_ w663] -> w634
          tunnel: w632 -> [_ w662]
          tunnel: w631 -> [w644 _]
          tunnel: w630 -> [w642 _]
          tunnel: w629 -> [_ w661]
          tunnel: w628 -> [_ w660]
          tunnel: w627 -> [_ w658]
          tunnel: w626 -> [_ w657]
          frame #0 {
            n158 = Merge Errors(w643, w644) -> (w641:errorcluster)
            n159 = local read "Archive Location"() -> (w649:path)
            n160 = call "Directory to Text file Compare FTP.vi"("error in (no error)"=w641, "delimiter (\\t)"="," ("delimiter (\\t)"), "File datastore Path IN"=w642, "File Pattern (*.CSV .ddf)"="*.ZIP", "Directory Path"=w649) -> ("Unmanaged Files"=w648:string[], "error out"=w640:errorcluster)  [unwired: 4 in, 1 out]
            n161 = for {
              tunnel: w648 -> [w656] mode=indexing
              tunnel: w647 -> [w655]
              tunnel: [w654] -> w646
              tunnel: [w653] -> w645
              tunnel: w640 -> [w652]
              n162 = Enqueue Element(queue=w655, element=w656, error in (no error)=w652) -> (queue out=w653:refnum<queue>, error out=w654:errorcluster)  [unwired: 1 in, 1 out]
            }
          }
          frame #1 {
            n163 = Get Queue Status(queue=w669, error in (no error)=w666) -> (queue out=w668:refnum<queue>, error out=w665:errorcluster, # elements in queue=w667:i32)  [unwired: 1 in, 5 out]
            n164 = Get Notifier Status(notifier=w660) -> (current notification=w659:bool)  [unwired: 1 in, 4 out]
            n165 = local read "Archive Location"() -> (w672:path)
            n166 = for {
              N: w667 -> [_]
              tunnel: [w692] -> w673
              tunnel: w670 -> [w690]
              tunnel: w672 -> [w678]
              tunnel: w668 -> [w691]
              tunnel: [w687] -> w671
              tunnel: [w689] -> w663
              tunnel: w665 -> [w685]
              tunnel: [w683] -> w664
              tunnel: w662 -> [w682]
              tunnel: w661 -> [w677]
              tunnel: w659 -> [w676]
              tunnel: w658 -> [w675]
              tunnel: w657 -> [w674]
              n167 = Dequeue Element(queue=w691, timeout in ms (-1)=5, error in (no error)=w685) -> (queue out=w688:refnum<queue>, element=w681:string, error out=w684:errorcluster)  [unwired: 1 out]
              n168 = call "FTP Move_Status_Errors.vi"("Active or Passive (Active = True)"=w675, "binary (F)"=w674, "Archived Path dir"=w678, "FTP input cluster"=w677, "Queue elements"=w681) -> ("concatenated string of Error"=w679:string, "ReQue element  errored"=w680:bool)  [unwired: 5 in]
              n169 = case shown="False" w676 {
                tunnel: [w703 w713] -> w692
                tunnel: w690 -> [w702 w712]
                tunnel: [w701 w712] -> w689
                tunnel: w688 -> [w700 w717]
                tunnel: [w699 w716] -> w687
                tunnel: w684 -> [w698 w715]
                tunnel: [w697 w714] -> w683
                tunnel: w682 -> [w696 w713]
                tunnel: w681 -> [w695 _]
                tunnel: w680 -> [w694 _]
                tunnel: w679 -> [w693 _]
                frame False {
                  n170 = case shown="False" w694 {
                    tunnel: w700 -> [w709 w711]
                    tunnel: w695 -> [w708 _]
                    tunnel: [w707 w711] -> w699
                    tunnel: w698 -> [w705 w710]
                    tunnel: [w704 w710] -> w697
                    frame False {
                      n171 = Enqueue Element(queue=w709, element=w708, timeout in ms (-1)=5, error in (no error)=w705) -> (queue out=w707:refnum<queue>, error out=w704:errorcluster)  [unwired: 1 out]
                    }
                    frame True {
                    }
                  }
                  n172 = Write to Text File(file (use dialog)=w696, text=w693, error in=w702) -> (refnum out=w703:refnum<file>, error out=w701:errorcluster)  [unwired: 1 in, 1 out]
                }
                frame True {
                  n173 = Flush Queue(queue=w717, error in (no error)=w715) -> (queue out=w716:refnum<queue>, error out=w714:errorcluster)  [unwired: 1 out]
                }
              }
            }
          }
        }
      }
      event Timeout {
        n174 = event-data() -> ()  [unwired: 1 in, 1 out]
        n175 = call "Timing 5min after 5min before.vi"() -> ("Mid Hour"=w723:bool)  [unwired: 5 in]
        n176 = case shown="True" w723 {
          tunnel: [w731 w745] -> w729
          tunnel: w728 -> [w733 w744]
          tunnel: [w733 w743] -> w727
          tunnel: w726 -> [w732 w742]
          tunnel: [w732 w741] -> w725
          tunnel: [w730 w740] -> w724
          tunnel: w722 -> [w731 w738]
          tunnel: w721 -> [w730 w737]
          tunnel: w720 -> [_ w736]
          tunnel: w719 -> [_ w735]
          tunnel: w718 -> [_ w734]
          frame False {
          }
          frame True {
            n177 = call "Elapsed Time2"() -> ("Time has Elapsed"=w739:bool)  [unwired: 12 in, 7 out]
            n178 = case shown="True" w739 {
              tunnel: [w746 w761] -> w745
              tunnel: w744 -> [w749 w760]
              tunnel: [w749 w759] -> w743
              tunnel: w742 -> [w748 w758]
              tunnel: [w748 w757] -> w741
              tunnel: [w747 w756] -> w740
              tunnel: w738 -> [w746 w754]
              tunnel: w737 -> [w747 w753]
              tunnel: w736 -> [_ w752]
              tunnel: w735 -> [_ w751]
              tunnel: w734 -> [_ w750]
              frame False {
              }
              frame True {
                n179 = stacked-sequence {
                  seq-local: [w768 _] -> [_ w789]
                  seq-local: [w767 _] -> [_ w788]
                  tunnel: [_ w792] -> w761
                  tunnel: w760 -> [w769 _]
                  tunnel: [_ w790] -> w759
                  tunnel: w758 -> [w766 w785]
                  tunnel: [_ w783] -> w757
                  tunnel: [_ w782] -> w756
                  tunnel: w754 -> [_ w781]
                  tunnel: w753 -> [w765 _]
                  tunnel: w752 -> [w764 _]
                  tunnel: w751 -> [_ w780]
                  tunnel: w750 -> [_ w779]
                  frame #0 {
                    n180 = local read "Archive Location"() -> (w771:path)
                    n181 = Merge Errors(w766, w765) -> (w763:errorcluster)
                    n182 = call "Directory to Text file Compare FTP.vi"("error in (no error)"=w763, "delimiter (\\t)"="," ("delimiter (\\t)"), "File datastore Path IN"=w764, "File Pattern (*.CSV .ddf)"="*.ZIP", "Directory Path"=w771) -> ("Unmanaged Files"=w770:string[], "error out"=w762:errorcluster)  [unwired: 4 in, 1 out]
                    n183 = for {
                      tunnel: w770 -> [w778] mode=indexing
                      tunnel: w769 -> [w777]
                      tunnel: [w776] -> w768
                      tunnel: [w775] -> w767
                      tunnel: w762 -> [w774]
                      n184 = Enqueue Element(queue=w777, element=w778, error in (no error)=w774) -> (queue out=w775:refnum<queue>, error out=w776:errorcluster)  [unwired: 1 in, 1 out]
                    }
                  }
                  frame #1 {
                    n185 = Get Queue Status(queue=w788, error in (no error)=w785) -> (queue out=w787:refnum<queue>, error out=w784:errorcluster, # elements in queue=w786:i32)  [unwired: 1 in, 5 out]
                    n186 = local read "Archive Location"() -> (w791:path)
                    n187 = for {
                      N: w786 -> [_]
                      tunnel: [w810] -> w792
                      tunnel: w789 -> [w809]
                      tunnel: w791 -> [w800]
                      tunnel: w787 -> [w795]
                      tunnel: [w806] -> w790
                      tunnel: [w808] -> w782
                      tunnel: w784 -> [w794]
                      tunnel: [w803] -> w783
                      tunnel: w781 -> [w802]
                      tunnel: w780 -> [w801]
                      tunnel: w779 -> [w796]
                      n188 = Get Notifier Status(notifier=w796) -> (current notification=w793:bool)  [unwired: 1 in, 4 out]
                      n189 = Dequeue Element(queue=w795, timeout in ms (-1)=5, error in (no error)=w794) -> (queue out=w807:refnum<queue>, element=w797:string, error out=w804:errorcluster)  [unwired: 1 out]
                      n190 = call "FTP Move_Status_Errors.vi"("Archived Path dir"=w800, "FTP input cluster"=w801, "Queue elements"=w797) -> ("concatenated string of Error"=w799:string, "ReQue element  errored"=w798:bool)  [unwired: 7 in]
                      n191 = case shown="False" w793 {
                        tunnel: [w821 w831] -> w810
                        tunnel: w809 -> [w820 w830]
                        tunnel: [w819 w830] -> w808
                        tunnel: w807 -> [w818 w835]
                        tunnel: [w817 w834] -> w806
                        tunnel: w804 -> [w816 w833]
                        tunnel: [w815 w832] -> w803
                        tunnel: w802 -> [w814 w831]
                        tunnel: w799 -> [w813 _]
                        tunnel: w798 -> [w812 _]
                        tunnel: w797 -> [w811 _]
                        frame False {
                          n192 = case shown="True" w812 {
                            tunnel: w818 -> [w827 w829]
                            tunnel: w811 -> [w826 _]
                            tunnel: [w825 w829] -> w817
                            tunnel: w816 -> [w823 w828]
                            tunnel: [w822 w828] -> w815
                            frame False {
                              n193 = Enqueue Element(queue=w827, element=w826, timeout in ms (-1)=5, error in (no error)=w823) -> (queue out=w825:refnum<queue>, error out=w822:errorcluster)  [unwired: 1 out]
                            }
                            frame True {
                            }
                          }
                          n194 = Write to Text File(file (use dialog)=w814, text=w813, error in=w820) -> (refnum out=w821:refnum<file>, error out=w819:errorcluster)  [unwired: 1 in, 1 out]
                        }
                        frame True {
                          n195 = Flush Queue(queue=w835, error in (no error)=w833) -> (queue out=w834:refnum<queue>, error out=w832:errorcluster)  [unwired: 1 out]
                        }
                      }
                    }
                  }
                }
                n196 = local write "Status FTP move"(TRUE ("Status FTP move")) -> ()
              }
            }
          }
        }
      }
    }
    n197 = Unbundle By Name("FTP Creds") -> ("Comp File Size"=w527:bool, "SITE ID"=w525:string)
    n198 = case shown="True" w527 {
      tunnel: w531 -> [w553 w560]
      tunnel: [w553 w559] -> w530
      tunnel: w529 -> [w552 w557]
      tunnel: [w552 w558] -> w528
      tunnel: "FTP Creds" -> [_ w556]
      tunnel: w525 -> [_ w554]
      frame False {
      }
      frame True {
        n199 = call "True at one time of day.vi"("Time stamp from INI (only will use time Not date)"="Time DaY") -> ("Time Until Next Scan (H)"=→"Elapsed Time (H)":dbl, "Time has Elapsed"=w561:bool)  [unwired: 8 in, 1 out]
        n200 = case shown="True" w561 {
          tunnel: w560 -> [w564 w578]
          tunnel: [w564 w580] -> w559
          tunnel: [w563 w579] -> w558
          tunnel: w557 -> [w563 w577]
          tunnel: w556 -> [_ w583]
          tunnel: w554 -> [_ w574]
          frame False {
          }
          frame True {
            w570 = "\r\n"
            n201 = local read "Archive Location"() -> (w581:path)
            n202 = call "Compare file size of FTP to Dir on local Machine.vi"("File Pattern (*.CSV .ddf)"="*.ZIP", "Local Path to compare file sizes to FTP"=w581, "FTP Creds"=w583) -> ("Equal File Sizes"=w576:cluster{"name":string, "Equal File size":bool}[])  [unwired: 7 in, 1 out]
            n203 = for {
              tunnel: [w594] -> w580
              tunnel: [w593] -> w579
              tunnel: w578 -> [w591]
              tunnel: w577 -> [w592]
              tunnel: w576 -> [w590] mode=indexing
              tunnel: [w587] -> w573 mode=indexing
              shift-right: [w585] -> w575
              shift-left: _ -> [w584]
              n204 = Unbundle By Name(w590) -> ("Equal File size"=w589:bool, "name"=w588:string)
              n205 = case shown="False" w589 {
                tunnel: [w600 w604] -> w594
                tunnel: [w599 w603] -> w593
                tunnel: w592 -> [w598 w603]
                tunnel: w591 -> [w597 w604]
                tunnel: w588 -> [w595 _]
                tunnel: [1 0] -> w586
                tunnel: [w595 ""] -> w587
                frame False {
                  n206 = Enqueue Element(queue=w597, element=w595, error in (no error)=w598) -> (queue out=w600:refnum<queue>, error out=w599:errorcluster)  [unwired: 1 in, 1 out]
                }
                frame True {
                }
              }
              n207 = Add(x=w584, y=w586) -> (x+y=w585:i32)
            }
            n208 = Concatenate Strings("FTP VS DIR File sizes are different at Site ID: " ("string"), w574) -> (w567:string)
            n209 = Concatenate Strings(w567, w570, "These files have been re-queued for FTP move agian, check to make sure files are up to date and moving correctly.\nFiles of issue are listed below.\n\nLIST:" ("string"), w570, w573) -> (w566:string)
            n210 = local read "Email Notification"() -> (w565:T3)
            n211 = local read "recipients"() -> (w568:string[])
            n212 = Greater Than 0?(x=w575) -> (x > 0?=w569:bool)
            n213 = call "Send Email Notification.vi"("Send Email Notification"=w569, "Mail Creds"=w565, "message"=w566, "Email Subject"=w567, "recipients"=w568) -> ()  [unwired: 7 in]
          }
        }
      }
    }
    n214 = Merge Errors(w528, w539) -> (w520:errorcluster)
    n215 = Unbundle By Name(w523) -> ("status"=w535:bool)
    n216 = case shown="Error" w520 {
      selector: w520 -> [w543 _]
      tunnel: [w543 errorcluster {"status"=FALSE, "code"=0, "source"=""} ("error IO")] -> w519
      frame No Error {
      }
      frame Error {
        n217 = local read "FTP Creds"() -> (w547:T2)
        n218 = Unbundle By Name(w547) -> ("SITE ID"=w546:string)
        n219 = local read "Email Notification"() -> (w549:T3)
        n220 = local read "recipients"() -> (w550:string[])
        n221 = Concatenate Strings("There was an Error with the FTP scan and Move at Site ID: " ("Email Subject"), w546) -> (w544:string)
        n222 = call "Send Email Notification.vi"("Send Email Notification"=TRUE, "Mail Creds"=w549, "message"=w544, "Email Subject"=w544, "recipients"=w550) -> ()  [unwired: 7 in]
      }
    }
    n223 = case shown="False" w535 {
      tunnel: [FALSE ("create directory if not found? (F)") TRUE ("create directory if not found? (F)")] -> w534
      frame False {
      }
      frame True {
        n224 = One Button Dialog(message="The File \"FTP FILE MOVE RECORD.CSV\" is open.\nPlease close the file before continuing.\n\nThis file is the log of past FTP movement and is needed by the software to maintain a history of already moved file. Please do not move or delete this file. This will result in unwanted actions by the software in attempt to send all files back up to the ftp again.\n") -> ()  [unwired: 1 in, 1 out]
      }
    }
  }
  n225 = while {
    shift-right: [w836] -> w111
    shift-left: w112 -> [w853]
    shift-right: [w841] -> w106
    shift-left: w68 -> [w844]
    tunnel: [w851] -> w228
    tunnel: [w850] -> w227
    tunnel: [w849] -> w226
    stop <- w842 stop-if-true
    n226 = local read "FTP Creds"() -> (w848:T2)
    n227 = local write "Status File move"(FALSE ("Status File move")) -> ()
    n228 = Equal?(x="Archive Location 2", y=path "") -> (x = y?=w861:bool)
    n229 = call <vilib>:"Check if File or Folder Exists.vi"("path"="Archive Location 2") -> ("file or folder exists?"=w860:bool, "dup path"=w856:path)  [unwired: 8 in, 1 out]
    n230 = Compound Arithmetic op=AND(w860, invert w861) -> (w857:bool)
    n231 = event shown="[0] Timeout" {
      selector: _ -> [_ _ _]
      dyn-events: _ -> [_ _ _]
      timeout: 30 -> [_ _ _]
      tunnel: w848 -> [w891 _ w996]
      tunnel: w857 -> [w890 _ w995]
      tunnel: w856 -> [w889 w974 w994]
      tunnel: "Archive Location" -> [w888 w975 w993]
      tunnel: "Rats Location" -> [w887 w976 w992]
      tunnel: w853 -> [w886 w972 w991]
      tunnel: [w885 w971 w990] -> w839
      tunnel: [w884 w976 w989] -> w851
      tunnel: [w883 w975 w988] -> w850
      tunnel: [w882 w974 w987] -> w849
      event Timeout {
        n232 = event-data() -> ()  [unwired: 1 in, 1 out]
        n233 = call "Timing 5min after 5min before.vi"() -> ("Mid Hour"=w881:bool)  [unwired: 5 in]
        n234 = case shown="True" w881 {
          tunnel: w887 -> [w896 w908]
          tunnel: w888 -> [w895 w907]
          tunnel: w889 -> [w894 w906]
          tunnel: w890 -> [_ w905]
          tunnel: w891 -> [w893 w903]
          tunnel: [w896 w902] -> w884
          tunnel: [w895 w901] -> w883
          tunnel: [w894 w900] -> w882
          tunnel: [w893 w899] -> _
          tunnel: w886 -> [w892 w898]
          tunnel: [w892 w897] -> w885
          frame False {
          }
          frame True {
            n235 = call "Elapsed Time"() -> ("Time has Elapsed"=w904:bool)  [unwired: 12 in, 7 out]
            n236 = case shown="True" w904 {
              tunnel: w908 -> [w913 w925]
              tunnel: w907 -> [w912 w924]
              tunnel: w906 -> [w911 w923]
              tunnel: w905 -> [_ w922]
              tunnel: w903 -> [w910 w921]
              tunnel: [w913 w920] -> w902
              tunnel: [w912 w919] -> w901
              tunnel: [w911 w918] -> w900
              tunnel: [w910 w917] -> w899
              tunnel: w898 -> [w909 w916]
              tunnel: [w909 w915] -> w897
              frame False {
              }
              frame True {
                n237 = stacked-sequence {
                  seq-local: [_ w938 _ _] -> [_ _ w952 _]
                  seq-local: [w933 _ _ _] -> [_ w944 _ _]
                  seq-local: [w932 _ _ _] -> [_ w937 _ _]
                  seq-local: [_ w941 _ _] -> [_ _ w950 _]
                  seq-local: [_ _ w949 _] -> [_ _ _ w966]
                  tunnel: w925 -> [w928 _ _ w970]
                  tunnel: w924 -> [w929 w945 w951 w969]
                  tunnel: w923 -> [w930 _ _ w968]
                  tunnel: w922 -> [w931 _ _ _]
                  tunnel: w921 -> [w927 _ _ w967]
                  tunnel: [_ _ _ w970] -> w920
                  tunnel: [_ _ _ w969] -> w919
                  tunnel: [_ _ _ w968] -> w918
                  tunnel: [_ _ _ w967] -> w917
                  tunnel: w916 -> [w926 _ _ _]
                  tunnel: [_ _ _ w966] -> w915
                  frame #0 {
                    n238 = Unbundle By Name(w927) -> ("Use ATL"=w936:bool)
                    n239 = Select(t="*.ATL" ("pattern"), s=w936, f="dont use the ALT files" ("pattern")) -> (s? t:f=w933:string)
                    n240 = call "File Move (incoming to Archive).vi"("Rats Location"=w928, "Archive Location"=w929, "Archive Location 2"=w930, "Archive 2 valid path"=w931, "error IO 2"=w926, "pattern"=w933) -> ("error IO"=w932:errorcluster)  [unwired: 9 in]
                  }
                  frame #1 {
                    n241 = call "Directory to list File compare.vi"("2nd File Type(s)(*.txt *.CSV)"="*.zip", "1st File Type(s)(*.txt *.CSV)"=w944, "error in (no error)"=w937, "2nd Directory (Zip)"=w945, "1st Directory (RATS)"=w945) -> ("error out"=w943:errorcluster, "Unmanaged Files"=w940:string[])  [unwired: 4 in, 1 out]
                    n242 = call "Directory to list File compare.vi"("2nd File Type(s)(*.txt *.CSV)"="*.zip", "1st File Type(s)(*.txt *.CSV)"="*.RAT" ("2nd File Type(s)(*.txt *.CSV)"), "error in (no error)"=w937, "2nd Directory (Zip)"=w945, "1st Directory (RATS)"=w945) -> ("error out"=w942:errorcluster, "Unmanaged Files"=w939:string[])  [unwired: 4 in, 1 out]
                    n243 = Insert Into Array(array=w940, new element=w939) -> (w938:string[])  [unwired: 1 in]
                    n244 = Merge Errors(w943, w942) -> (w941:errorcluster)
                  }
                  frame #2 {
                    n245 = for {
                      tunnel: w952 -> [w954] mode=indexing
                      tunnel: w951 -> [w953]
                      shift-right: [w959] -> w949
                      shift-left: w950 -> [w960]
                      n246 = Build Path(base path=w953, name or relative path=w954) -> (appended path=w957:path)
                      n247 = String To Path(string=w954) -> (path=w961:path)
                      n248 = Concatenate Strings(w954, ".Zip" ("name or relative path")) -> (w955:string)
                      n249 = Build Path(base path=w953, name or relative path=w955) -> (appended path=w958:path)
                      n250 = call <vilib>:"New Zip File.vi"("error in (no error)"=w960, "target"=w958) -> ("error out"=w962:errorcluster, "zip file out"=w965:i64)  [unwired: 3 in, 1 out]
                      n251 = call <vilib>:"Add File to Zip.vi"("error in (no error)"=w962, "destination path in zip"=w961, "source file path"=w957, "zip file in"=w965) -> ("error out"=w964:errorcluster, "zip file out"=w963:i64)  [unwired: 6 in]
                      n252 = call <vilib>:"Close Zip File.vi"("error in (no error)"=w964, "zip file in"=w963) -> ("error out"=w959:errorcluster)  [unwired: 5 in]
                    }
                  }
                  frame #3 {
                  }
                }
                n253 = local write "Status File move"(TRUE ("Status File move")) -> ()
              }
            }
          }
        }
      }
      event Menu Selection (User) {
        n254 = event-data() -> ("ItemTag"=w977:string)  [unwired: 1 in]
        n255 = case shown="\"Exit\"" w977 {
          tunnel: [errorcluster {"status"=FALSE, "code"=0, "source"=""} ("error out") w979 errorcluster {"status"=FALSE, "code"=0, "source"=""} ("error out")] -> w973
          frame "Null", Default {
          }
          frame "Exit" {
            n256 = Obtain Notifier(name (unnamed)="Shutdown", notification data type=TRUE) -> (notifier out=w982:refnum<notifier>, error out=w984:errorcluster)  [unwired: 2 in, 1 out]
            n257 = Send Notification(notification=TRUE, notifier=w982, error in (no error)=w984) -> (error out=w979:errorcluster)  [unwired: 1 out]
          }
          frame "NAF" {
            n258 = call "About.vi"() -> ()  [unwired: 12 in]
          }
        }
        n259 = Merge Errors(w973, w972) -> (w971:errorcluster)
      }
      event "Manual Archive": Value Change {
        n260 = event-data() -> ()  [unwired: 1 in, 1 out]
        n261 = stacked-sequence {
          seq-local: [_ w1009 _ _] -> [_ _ w1023 _]
          seq-local: [w1004 _ _ _] -> [_ w1015 _ _]
          seq-local: [w1003 _ _ _] -> [_ w1008 _ _]
          seq-local: [_ w1012 _ _] -> [_ _ w1021 _]
          seq-local: [_ _ w1020 _] -> [_ _ _ w1037]
          tunnel: w992 -> [w999 _ _ w1040]
          tunnel: w993 -> [w1000 w1016 w1022 w1039]
          tunnel: w994 -> [w1001 _ _ w1038]
          tunnel: w995 -> [w1002 _ _ _]
          tunnel: w996 -> [w998 _ _ _]
          tunnel: [_ _ _ w1040] -> w989
          tunnel: [_ _ _ w1039] -> w988
          tunnel: [_ _ _ w1038] -> w987
          tunnel: w991 -> [w997 _ _ _]
          tunnel: [_ _ _ w1037] -> w990
          frame #0 {
            n262 = Unbundle By Name(w998) -> ("Use ATL"=w1007:bool)
            n263 = Select(t="*.ATL" ("pattern"), s=w1007, f="dont use the ALT files" ("pattern")) -> (s? t:f=w1004:string)
            n264 = call "File Move (incoming to Archive).vi"("Rats Location"=w999, "Archive Location"=w1000, "Archive Location 2"=w1001, "Archive 2 valid path"=w1002, "error IO 2"=w997, "pattern"=w1004) -> ("error IO"=w1003:errorcluster)  [unwired: 9 in]
          }
          frame #1 {
            n265 = call "Directory to list File compare.vi"("2nd File Type(s)(*.txt *.CSV)"="*.zip", "1st File Type(s)(*.txt *.CSV)"=w1015, "error in (no error)"=w1008, "2nd Directory (Zip)"=w1016, "1st Directory (RATS)"=w1016) -> ("error out"=w1014:errorcluster, "Unmanaged Files"=w1011:string[])  [unwired: 4 in, 1 out]
            n266 = call "Directory to list File compare.vi"("2nd File Type(s)(*.txt *.CSV)"="*.zip", "1st File Type(s)(*.txt *.CSV)"="*.RAT" ("2nd File Type(s)(*.txt *.CSV)"), "error in (no error)"=w1008, "2nd Directory (Zip)"=w1016, "1st Directory (RATS)"=w1016) -> ("error out"=w1013:errorcluster, "Unmanaged Files"=w1010:string[])  [unwired: 4 in, 1 out]
            n267 = Insert Into Array(array=w1011, new element=w1010) -> (w1009:string[])  [unwired: 1 in]
            n268 = Merge Errors(w1014, w1013) -> (w1012:errorcluster)
          }
          frame #2 {
            n269 = for {
              tunnel: w1023 -> [w1025] mode=indexing
              tunnel: w1022 -> [w1024]
              shift-right: [w1030] -> w1020
              shift-left: w1021 -> [w1031]
              n270 = Build Path(base path=w1024, name or relative path=w1025) -> (appended path=w1028:path)
              n271 = String To Path(string=w1025) -> (path=w1032:path)
              n272 = Concatenate Strings(w1025, ".Zip" ("name or relative path")) -> (w1026:string)
              n273 = Build Path(base path=w1024, name or relative path=w1026) -> (appended path=w1029:path)
              n274 = call <vilib>:"New Zip File.vi"("error in (no error)"=w1031, "target"=w1029) -> ("error out"=w1033:errorcluster, "zip file out"=w1036:i64)  [unwired: 3 in, 1 out]
              n275 = call <vilib>:"Add File to Zip.vi"("error in (no error)"=w1033, "destination path in zip"=w1032, "source file path"=w1028, "zip file in"=w1036) -> ("error out"=w1035:errorcluster, "zip file out"=w1034:i64)  [unwired: 6 in]
              n276 = call <vilib>:"Close Zip File.vi"("error in (no error)"=w1035, "zip file in"=w1034) -> ("error out"=w1030:errorcluster)  [unwired: 5 in]
            }
          }
          frame #3 {
          }
        }
        n277 = local write "Status File move"(TRUE ("Status File move")) -> ()
      }
    }
    n278 = case shown="False" "ShutDown" {
      tunnel: [FALSE ("Status File move") w879] -> w845
      frame False {
      }
      frame True {
        n279 = Two Button Dialog(message="Are you sure you want to shut down NODE ARCHIVE & FTP? This will end all file management of the Archive directories and FTP file movement until the software is restarted.\nIf the Archiving In Progress, or the FTP In Progress is lit the software will shut down as soon as the process is done.", 2:"Shutdown" ("T button name (\"OK\")")) -> (T button?=w879:bool)  [unwired: 1 in]
      }
    }
    n280 = case shown="False" w845 {
      tunnel: w844 -> [w863 w866]
      tunnel: [w863 w865] -> w843
      tunnel: [errorcluster {"status"=FALSE, "code"=0, "source"=""} ("error out") w864] -> w840
      frame False {
      }
      frame True {
        n281 = Send Notification(notification=TRUE, notifier=w866) -> (notifier out=w865:refnum<notifier>, error out=w864:errorcluster)  [unwired: 1 in]
      }
    }
    n282 = Get Notifier Status(notifier=w843, error in (no error)=w840) -> (notifier out=w841:refnum<notifier>, current notification=w842:bool, error out=w838:errorcluster)  [unwired: 2 out]
    n283 = Merge Errors(w839, w838) -> (w837:errorcluster)
    n284 = case shown="No Error" w837 {
      selector: w837 -> [w868 _]
      tunnel: [w868 errorcluster {"status"=FALSE, "code"=0, "source"=""} ("error IO")] -> w836
      frame No Error {
      }
      frame Error {
        n285 = local read "FTP Creds"() -> (w872:T2)
        n286 = Unbundle By Name(w872) -> ("SITE ID"=w871:string)
        n287 = local read "Email Notification"() -> (w874:T3)
        n288 = local read "recipients"() -> (w875:string[])
        n289 = Concatenate Strings("Archiving and Zipping  at Site: " ("Email Subject"), w871) -> (w869:string)
        n290 = call "Send Email Notification.vi"("Send Email Notification"=TRUE, "Mail Creds"=w874, "message"=w869, "Email Subject"=w869, "recipients"=w875) -> ()  [unwired: 7 in]
      }
    }
  }
  n291 = call <vilib>:"Get System Directory.vi"("create directory if not found? (F)"=TRUE, "system directory type"=w155) -> ("system directory"=w154:path)  [unwired: 9 in]
  n292 = Build Path(base path=w154, name or relative path="Logs\\" ("string")) -> (appended path=w158:path)
  n293 = Create Folder(path (use dialog)=w158) -> (created path=w159:path)  [unwired: 2 in, 2 out]
  n294 = Build Path(base path=w159, name or relative path="Node FTP and STATS.INI") -> (appended path=w153:path)
  n295 = call <vilib>:"Open Config Data.vi"("create file if necessary (T)"=TRUE, "configuration file path"=w153) -> ("error out"=w243:errorcluster, "refnum"=w244:T6)  [unwired: 7 in, 1 out]
  n296 = call-poly <vilib>:"Write Key.vi"("section"=w250, "error in (no error)"=w243, "value"=w228, "key"="Rat Locations" ("name or relative path"), "refnum"=w244) -> ("error out"=w246:errorcluster, "refnum out"=w245:T6)  [unwired: 4 in, 1 out]
  n297 = call-poly <vilib>:"Write Key.vi"("section"=w250, "error in (no error)"=w246, "value"=w227, "key"="Archive" ("name or relative path"), "refnum"=w245) -> ("error out"=w248:errorcluster, "refnum out"=w247:T6)  [unwired: 4 in, 1 out]
  n298 = call-poly <vilib>:"Write Key.vi"("section"=w250, "error in (no error)"=w248, "value"=w226, "key"="Archive 2" ("name or relative path"), "refnum"=w247) -> ("error out"=w254:errorcluster, "refnum out"=w260:T6)  [unwired: 4 in, 1 out]
  n299 = Unbundle By Name(w175) -> ("Host"=w241:string, "UserName"=w240:string, "PassWord"=w239:string, "FTP File Path"=w238:string, "FTP Timeout (S)"=w237:i32, "Use ATL"=w236:bool, "Comp File Size"=w197:bool, "SITE ID"=w176:string)
  n300 = call-poly <vilib>:"Write Key.vi"("section"=w266, "error in (no error)"=w254, "value"=w241, "key"="Host" ("name or relative path"), "refnum"=w260) -> ("error out"=w255:errorcluster, "refnum out"=w261:T6)  [unwired: 4 in, 1 out]
  n301 = call-poly <vilib>:"Write Key.vi"("section"=w266, "error in (no error)"=w255, "value"=w240, "key"="UserName" ("name or relative path"), "refnum"=w261) -> ("error out"=w256:errorcluster, "refnum out"=w262:T6)  [unwired: 4 in, 1 out]
  n302 = call-poly <vilib>:"Write Key.vi"("section"=w266, "error in (no error)"=w256, "value"=w239, "key"="Password" ("name or relative path"), "refnum"=w262) -> ("error out"=w257:errorcluster, "refnum out"=w263:T6)  [unwired: 4 in, 1 out]
  n303 = Merge Errors(w168, w127, w126) -> (w167:errorcluster)
  n304 = call-poly <vilib>:"Write Key.vi"("section"=w266, "error in (no error)"=w257, "value"=w238, "key"="FTP File Path" ("name or relative path"), "refnum"=w263) -> ("error out"=w258:errorcluster, "refnum out"=w264:T6)  [unwired: 4 in, 1 out]
  n305 = call-poly <vilib>:"Write Key.vi"("section"=w266, "error in (no error)"=w258, "value"=w237, "key"="FTP Timeout" ("name or relative path"), "refnum"=w264) -> ("error out"=w259:errorcluster, "refnum out"=w265:T6)  [unwired: 4 in, 1 out]
  n306 = call-poly <vilib>:"Write Key.vi"("section"=w266, "error in (no error)"=w259, "value"=w236, "key"="Archive Zip .ATL" ("name or relative path"), "refnum"=w265) -> ("error out"=w205:errorcluster, "refnum out"=w204:T6)  [unwired: 4 in, 1 out]
  n307 = call-poly <vilib>:"Write Key.vi"("section"=w201, "error in (no error)"=w205, "value"=w196, "key"="File size Compare (FTP to DIR)" ("name or relative path"), "refnum"=w204) -> ("error out"=w203:errorcluster, "refnum out"=w202:T6)  [unwired: 4 in, 1 out]
  n308 = Release Queue(queue=w206, error in (no error)=w101) -> (error out=w102:errorcluster)  [unwired: 1 in, 2 out]
  n309 = Close File(refnum=w225, error in=w100) -> (error out=w103:errorcluster)  [unwired: 1 out]
  n310 = call-poly <vilib>:"Write Key.vi"("section"=w201, "error in (no error)"=w203, "value"=w197, "key"="Use File size Compare (FTP to DIR)" ("name or relative path"), "refnum"=w202) -> ("error out"=w180:errorcluster, "refnum out"=w179:T6)  [unwired: 4 in, 1 out]
  n311 = Unbundle By Name(w83) -> ("AddressNode 1"=w72:string, "AddressNode2"=w71:string, "Addresshost"=w70:string)
  n312 = call-poly <vilib>:"Write Key.vi"("section"="SITE" ("name or relative path"), "error in (no error)"=w180, "value"=w176, "key"="Site ID" ("name or relative path"), "refnum"=w179) -> ("error out"=w75:errorcluster, "refnum out"=w76:T6)  [unwired: 4 in, 1 out]
  n313 = Merge Errors(w102, w103, w167) -> (w220:errorcluster)
  n314 = call-poly <vilib>:"Write Key.vi"("section"=w80, "error in (no error)"=w75, "value"=w72, "key"="Node 1" ("Mail Server"), "refnum"=w76) -> ("error out"=w74:errorcluster, "refnum out"=w81:T6)  [unwired: 4 in, 1 out]
  n315 = call-poly <vilib>:"Write Key.vi"("section"=w80, "error in (no error)"=w74, "value"=w71, "key"="Node 2" ("Mail Server"), "refnum"=w81) -> ("error out"=w73:errorcluster, "refnum out"=w82:T6)  [unwired: 4 in, 1 out]
  n316 = call-poly <vilib>:"Write Key.vi"("section"=w80, "error in (no error)"=w73, "value"=w70, "key"="FTP Host" ("Mail Server"), "refnum"=w82) -> ("error out"=w14:errorcluster, "refnum out"=w15:T6)  [unwired: 4 in, 1 out]
  n317 = Unbundle By Name(w11) -> ("Mail Server"=w10:string, "Return Address"=w9:string, "Email User Name"=w8:string, "Password"=w7:string)
  n318 = call-poly <vilib>:"Write Key.vi"("section"=w2, "error in (no error)"=w14, "value"=w10, "key"="Mail Server" ("Mail Server"), "refnum"=w15) -> ("error out"=w20:errorcluster, "refnum out"=w21:T6)  [unwired: 4 in, 1 out]
  n319 = call-poly <vilib>:"Write Key.vi"("section"=w2, "error in (no error)"=w20, "value"=w9, "key"="Return Address" ("Return Address"), "refnum"=w21) -> ("error out"=w22:errorcluster, "refnum out"=w25:T6)  [unwired: 4 in, 1 out]
  n320 = call-poly <vilib>:"Write Key.vi"("section"=w2, "error in (no error)"=w22, "value"=w8, "key"="User Name" ("Email User Name"), "refnum"=w25) -> ("error out"=w23:errorcluster, "refnum out"=w24:T6)  [unwired: 4 in, 1 out]
  n321 = call-poly <vilib>:"Write Key.vi"("section"=w2, "error in (no error)"=w23, "value"=w7, "key"="Password" ("Password"), "refnum"=w24) -> ("error out"=w28:errorcluster, "refnum out"=w27:T6)  [unwired: 4 in, 1 out]
  n322 = Array To Spreadsheet String(delimiter (Tab)=",", array=w6, 3:"%s" ("format string")) -> (spreadsheet string=w3:string)
  n323 = call-poly <vilib>:"Write Key.vi"("section"=w2, "error in (no error)"=w28, "value"=w3, "key"="Email_Recipients" ("Password"), "refnum"=w27) -> ("error out"=w12:errorcluster, "refnum out"=w13:T6)  [unwired: 4 in, 1 out]
  n324 = call <vilib>:"Close Config Data.vi"("error in (no error)"=w12, "write file if changed (T)"=TRUE, "refnum"=w13) -> ("error out"=w148:errorcluster)  [unwired: 7 in, 1 out]
  n325 = case shown="Error" w148 {
    selector: w148 -> [w1041 _]
    tunnel: [w1041 errorcluster {"status"=FALSE, "code"=0, "source"=""} ("error IO")] -> w69
    frame No Error {
    }
    frame Error {
      w1045 = T7 4 items=["no dialog", "OK message", "continue or stop message", "OK message + warnings", "continue/stop + warnings"] ("type of dialog (OK msg:1)")
      n326 = call <vilib>:"Simple Error Handler.vi"("error code (no error:0)"=5002, "error source (\" \")"="Writing values to the INI File" ("error source (\" \")"), "type of dialog (OK msg:1)"=w1045) -> ()  [unwired: 2 in, 5 out]
    }
  }
  n327 = Merge Errors(w69, w111, w220) -> (w107:errorcluster)
  n328 = Release Notifier(notifier=w106, force destroy? (F)=TRUE, error in (no error)=w107) -> (error out=w109:errorcluster)  [unwired: 2 out]
  n329 = call <vilib>:"Clear Errors.vi"("error in (no error)"=w109) -> ("error out"=w108:errorcluster)  [unwired: 6 in]
  n330 = property class="App"(error in=w108) -> (error out=w110:errorcluster, "App.Kind"=w221:T10)  [unwired: 1 in, 1 out]
  n331 = case shown="\"Run Time System\"" w221 {
    tunnel: w110 -> [_ _ _ _ _ _ _]
    frame "invalid app kind", Default {
    }
    frame "Development System" {
    }
    frame "Run Time System" {
      n332 = Quit LabVIEW() -> ()  [unwired: 1 in]
    }
    frame "Student Edition" {
    }
    frame "Embedded LabVIEW" {
    }
    frame "Evaluation" {
    }
    frame "Custom" {
    }
  }
  "Status File move" <- FALSE ("Status File move")
  "Status FTP move" <- FALSE ("Status FTP move")
